vi "Check Connection.vi"(3 "error In":errorcluster, 4 "State In":enum16{"Not Connected", "Init", "Connected"}(ring), 5 "VI reference":refnum<vi>) -> (0 "error out":errorcluster, 1 "State Out":enum16{"Not Connected", "Init", "Connected"}(ring), 2 "dup VI reference":refnum<vi>)   [LabVIEW 2021]
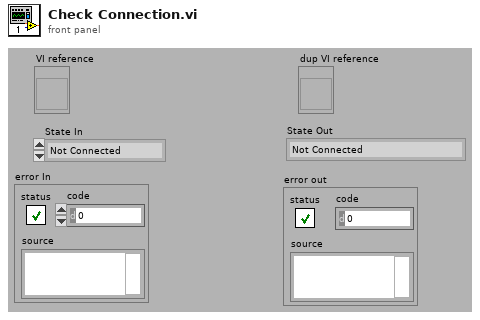
[diagram p1: front panel]
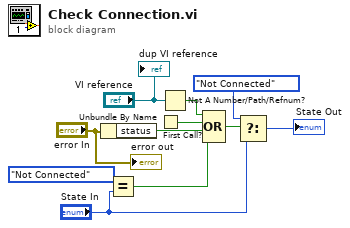
[diagram p0: block diagram]
diagram:
  n1 = Unbundle By Name("error In") -> ("status"=w9:bool)
  n2 = Equal?(x=enum16{"Not Connected", "Init", "Connected"}."Not Connected" ("y"), y="State In") -> (x = y?=w8:bool)
  n3 = First Call?() -> (First Call?: T/F=w11:bool)
  n4 = Not A Number/Path/Refnum?(number/path/refnum="VI reference") -> (NaN/Path/Refnum?=w10:bool)
  n5 = Compound Arithmetic op=OR(w10, w11, w9, w8) -> (w7:bool)
  n6 = Select(t=enum16{"Not Connected", "Init", "Connected"}."Not Connected" ("y"), s=w7, f="State In") -> (s? t:f=→"State Out":enum16{"Not Connected", "Init", "Connected"})
  "error out" <- "error In"
  "dup VI reference" <- "VI reference"
